vi "configure.vi"(8 "error in (no error)":errorcluster, 9 "timeStamp":string, 10 "Path":path, 11 "HWController in":refnum<class "HWController.lvclass">) -> (0 "error out":errorcluster, 3 "HWController out":refnum<class "HWController.lvclass">)   [LabVIEW 2009, in "Hardware.lvlib" / "HWControllers.lvlib" / "HWController.lvclass"]
uses:
  HWController.lvclass
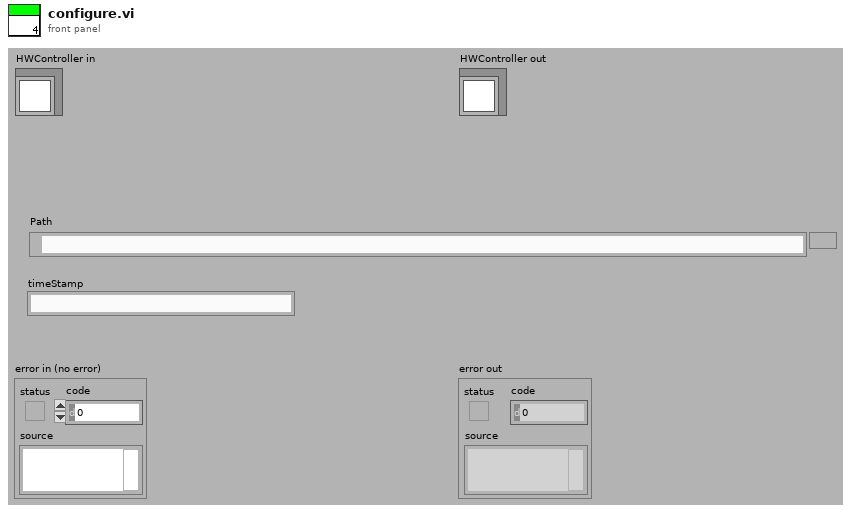
[diagram p1: front panel]
types:
  T1 = enum16{"Ready", "Compiling", "Configured", "Running", "Stopping", "Unresolved Error"}
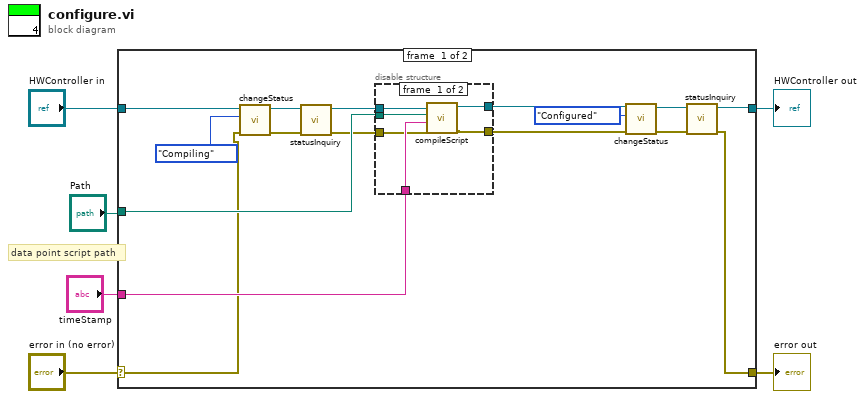
[diagram p0: block diagram]
diagram:
  # "data point script path"
  n1 = case shown="No Error" "error in (no error)" {
    selector: "error in (no error)" -> [w8 w32]
    tunnel: [w19 w32] -> w5
    tunnel: [w20 w31] -> w3
    tunnel: "HWController in" -> [w9 w31]
    tunnel: "Path" -> [w17 _]
    tunnel: "timeStamp" -> [w16 _]
    frame #0 {
      n2 = call "changeStatus.vi"("error in (no error)"=w8, "status"=T1."Compiling", "HWController in"=w9) -> ("error out"=w13:errorcluster, "HWController out"=w12:refnum<class "HWController.lvclass">)  [unwired: 7 in]
      n3 = call-dynamic "statusInquiry.vi"("error in (no error)"=w13, "HWController in"=w12) -> ("error out"=w7:errorcluster, "HWController out"=w10:refnum<class "HWController.lvclass">)  [unwired: 8 in]
      n4 = disable-structure shown="Enabled" {
        disable-tunnel: [w28 w30] -> w18
        disable-tunnel: w17 -> [w27 _]
        disable-tunnel: w16 -> [w26 _]
        disable-tunnel: [w25 w29] -> w15
        disable-tunnel: w10 -> [w24 w30]
        disable-tunnel: w7 -> [w23 w29]
        frame #0 {
          n5 = call "compileScript.vi"("error in (no error)"=w23, "timeStamp"=w26, "Path"=w27, "HWController in"=w24) -> ("error out"=w25:errorcluster, "HWController out"=w28:refnum<class "HWController.lvclass">)  [unwired: 4 in, 2 out]
        }
        frame #1 {
        }
      }
      n6 = call "changeStatus.vi"("error in (no error)"=w15, "status"=T1."Configured", "HWController in"=w18) -> ("error out"=w22:errorcluster, "HWController out"=w21:refnum<class "HWController.lvclass">)  [unwired: 7 in]
      n7 = call-dynamic "statusInquiry.vi"("error in (no error)"=w22, "HWController in"=w21) -> ("error out"=w19:errorcluster, "HWController out"=w20:refnum<class "HWController.lvclass">)  [unwired: 8 in]
    }
    frame #1 {
    }
  }
  "error out" <- w5
  "HWController out" <- w3
